vi "EnableControls.vi"(8 "error in (no error)":errorcluster, 10 "event data":cluster{"Label":string, "Visable?":bool}, 11 "OxxiusLaserController in":refnum<class "LaserController.lvclass">) -> (0 "error out":errorcluster, 3 "OxxiusLaserController out":refnum<class "LaserController.lvclass">)   [LabVIEW 2020, in "LaserController.lvlib" / "LaserController.lvclass"]
uses:
  LaserController.lvclass
  LaserController.lvclass/LaserController.ctl
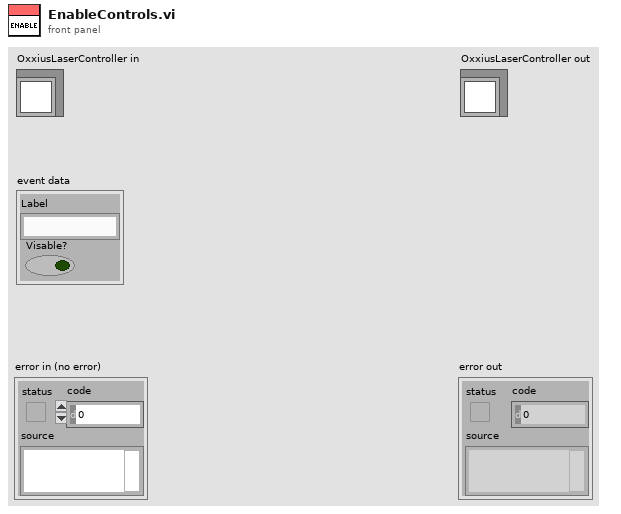
[diagram p1: front panel]
types:
  T1 = map{string, cluster{"Status":refnum<vi>, "Auto":refnum<vi>, "Power":refnum<vi>}}
  T2 = cluster{"Status":refnum<vi>, "Auto":refnum<vi>, "Power":refnum<vi>}
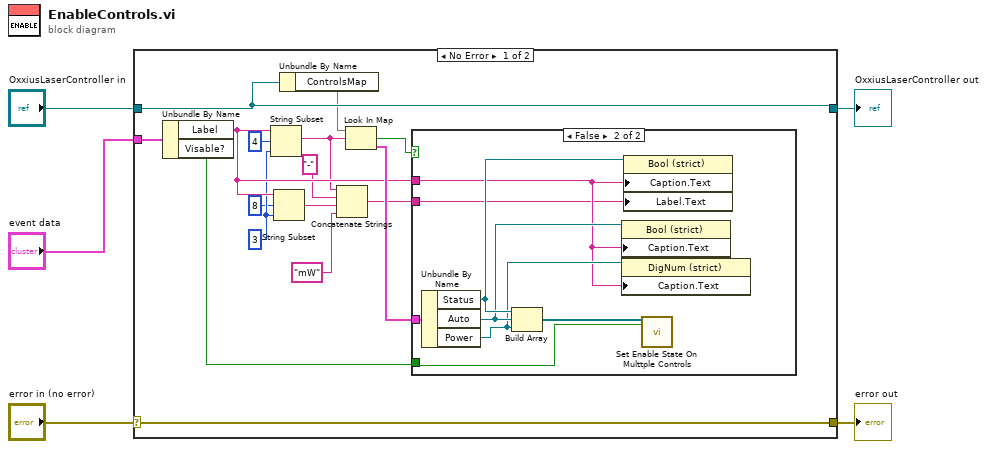
[diagram p0: block diagram]
diagram:
  n1 = case shown="No Error" "error in (no error)" {
    selector: "error in (no error)" -> [w21 w31]
    tunnel: [w21 w31] -> w4
    tunnel: [w17 w30] -> w2
    tunnel: "OxxiusLaserController in" -> [w17 w30]
    tunnel: "event data" -> [w18 _]
    frame No Error {
      w12 = 3 ("length (rest)")
      n2 = Unbundle By Name(w18) -> ("Label"=w13:string, "Visable?"=w20:bool)
      n3 = String Subset(string=w13, offset (0)=4, length (rest)=w12) -> (substring=w10:string)
      n4 = String Subset(string=w13, offset (0)=8, length (rest)=w12) -> (substring=w9:string)
      n5 = Unbundle By Name(w17) -> ("ControlsMap"=w16:T1)
      n6 = Concatenate Strings(w10, "-" ("string"), w9, "mW" ("string")) -> (w6:string)
      n7 = Look In Map(map=w16, key=w10) -> (key not found?=w14:bool, value=w15:T2)  [unwired: 1 in]
      n8 = case shown="False" w14 {
        tunnel: w20 -> [_ w28]
        tunnel: w15 -> [_ w27]
        tunnel: w13 -> [_ w23]
        tunnel: w6 -> [_ w22]
        frame True {
        }
        frame False {
          n9 = Unbundle By Name(w27) -> ("Status"=w26:refnum<vi>, "Auto"=w25:refnum<vi>, "Power"=w24:refnum<vi>)
          n10 = Build Array(w26, w25, w24) -> (w29:refnum<vi>[])
          n11 = property class="Bool (strict)"(reference=w25, "Caption.Text"=w23) -> ()  [unwired: 1 in, 2 out]
          n12 = property class="DigNum (strict)"(reference=w24, "Caption.Text"=w23) -> ()  [unwired: 1 in, 2 out]
          n13 = property class="Bool (strict)"(reference=w26, "Caption.Text"=w23, "Label.Text"=w22) -> ()  [unwired: 1 in, 2 out]
          n14 = call "Set Enable State On Multtple Controls.vi"("Controls"=w29, "Enable?"=w28) -> ()  [unwired: 18 in]
        }
      }
    }
    frame Error {
    }
  }
  "error out" <- w4
  "OxxiusLaserController out" <- w2
